vi "Get Temporary String Property.vi"(8 "error in (no error)":errorcluster, 10 "property name":string, 11 "Item Ref in":T1 format="%.0x") -> (0 "error out":errorcluster, 2 "value":string, 3 "Item Ref out":T1 format="%.0x", 4 "found?":bool)   [LabVIEW 2020, in "Routing and Faulting System Explorer.lvlib"]
uses:
  Routing and Faulting System Explorer.lvlib
  <vilib>/NI VeriStand/Custom Device API/Custom Device Item Ref.ctl
  NationalInstruments.VeriStand.SystemStorage
  Scripting/Routing and Faulting Scripting.lvlib
  <vilib>/NI VeriStand/Custom Device API/Custom Device API.lvlib
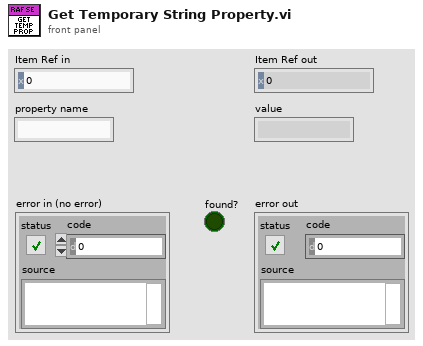
[diagram p1: front panel]
types:
  T1 = typedef "Custom Device API.lvlib/Custom Device Item Ref.ctl" = u64
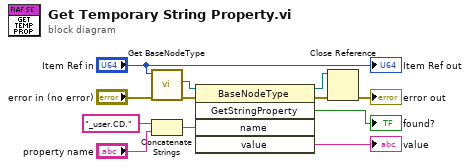
[diagram p0: block diagram]
diagram:
  n1 = call "Get BaseNodeType.vi"("error in"="error in (no error)", "item in"="Item Ref in") -> ("error out"=w4:errorcluster, "BaseNodeType"=w10:refnum<k24>)  [unwired: 7 in, 1 out]
  n2 = Concatenate Strings("_user.CD." ("string"), "property name") -> (w9:string)
  n3 = invoke class="BaseNodeType" method="GetStringProperty"(reference=w10, error in=w4, "name"=w9) -> (reference out=w6:refnum<k24>, error out=w7:errorcluster, "GetStringProperty"=→"found?":bool, "value"=→"value":string)  [unwired: 2 in, 1 out]
  n4 = Close Reference(reference=w6, error in (no error)=w7) -> (error out=→"error out":errorcluster)
  "Item Ref out" <- "Item Ref in"
